vi "Subvi buffer input LUT.vi"(2 "Buffer":refnum<k21>="GALVO1") -> ()   [LabVIEW 2017]
uses:
  GV FIFOIN timeout.vi
  <vilib>/rvi/interface/RandomDataEmulation/niFpgaRandomDataHandleErrors.vi
  <vilib>/rvi/DataTransferAndStorage/Container/Common/niFpgaContainerExecOnDevCompGetState.vi
  <vilib>/rvi/Emulation/niFpgaEmulationIsFPGAContextNoSignature.vi
  <vilib>/rvi/DataTransferAndStorage/Container/Common/niFpgaContainerGetUniqueNameForEmu.vi
  <vilib>/rvi/Emulation/niFpgaProcessEmulError.vi
  <vilib>/rvi/Emulation/niFpgaSctlEmulationGetInTimedLoop.vi
  <vilib>/rvi/errors/nirviReportUnexpectedCaseInternalError (U32).vi
  <vilib>/rvi/Memory/Memory_Emulation/niFpgaMemoryEmulationCacheClearOnFirstRun.vi
  <vilib>/rvi/Memory/Memory_Emulation/nirvimemoryEmulationManagerCache_MakeExclusive.vi
  <vilib>/rvi/Memory/Memory_Emulation/niFpgaMemoryEmulationValidateCache.vi
  <vilib>/rvi/Memory/Memory_Emulation/nirvimemoryEmulationManagerCache_InsertValue.vi
  <vilib>/Utility/error.llb/Clear Errors.vi
  <vilib>/rvi/Memory/Memory_Emulation/nirvimemoryEmulationManagerCache_ReleaseExclusive.vi
  <vilib>/rvi/Memory/Memory_Emulation/nirvimemoryEmulationManagerCache_GetValue.vi
  <vilib>/rvi/Memory/Memory_Emulation/nirvimemoryEmulationManagerCache_SetValue.vi
  <vilib>/rvi/Emulation/niFpgaSctlEmulationResourceMgr.vi
  <vilib>/rvi/DataTransferAndStorage/Container/XNode/niFpgaContainer.xnode
  <vilib>/rvi/interface/RandomDataEmulation/nirviRandomDataFpgaReadWriteTemplate.vi
  <vilib>/rvi/Memory/Memory_Emulation/niFpgaMemoryEmulationRefIn.vi
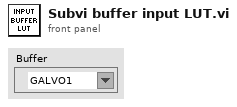
[diagram p1: front panel]
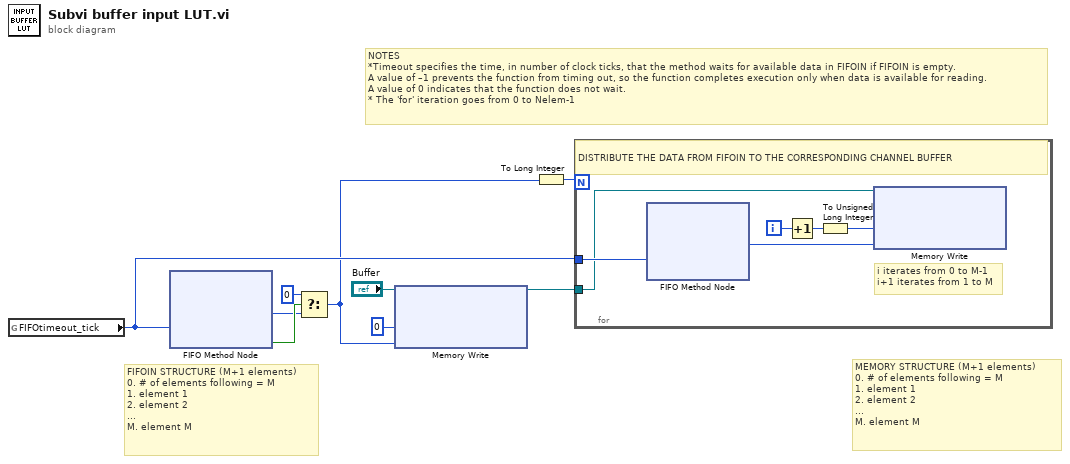
[diagram p0: block diagram]
diagram:
  # "MEMORY STRUCTURE (M+1 elements)\n0. # of elements following = M\n1. element 1\n2. element 2\n...\nM. element M"
  # "FIFOIN STRUCTURE (M+1 elements)\n0. # of elements following = M\n1. element 1\n2. element 2\n...\nM. element M"
  # "NOTES\n*Timeout specifies the time, in number of clock ticks, that the method waits for available data in FIFOIN if FIFOIN is empty.\nA value of –1 prevents the function from timing out, so the function completes execution only when data is available for reading.\nA value of 0 indicates that the function does not wait.\n* The 'for' iteration goes from 0 to Nelem-1"
  n1 = global read "GV FIFOIN timeout.vi" "FIFOtimeout_tick"() -> (w7:i32)
  n2 = xnode ("FIFO Method Node")("Timeout"=w7) -> ("Element"=w5:u32, "Timed Out?"=w6:bool)  [unwired: 1 in, 1 out]
  n3 = Select(t=u32 0, s=w6, f=w5) -> (s? t:f=w3:u32)
  n4 = xnode ("Memory Write")("Address"=u32 0, "Data"=w3, "Memory In"="Buffer") -> ("Memory Out"=w2:refnum<k21>)
  n5 = To Long Integer(number=w3) -> (32bit integer=w8:i32)
  n6 = for {
    N: w8 -> [_]
    tunnel: w7 -> [w15]
    tunnel: w2 -> [w12]
    i -> [w14]
    # "i iterates from 0 to M-1\ni+1 iterates from 1 to M"
    # "DISTRIBUTE THE DATA FROM FIFOIN TO THE CORRESPONDING CHANNEL BUFFER"
    n7 = xnode ("FIFO Method Node")("Timeout"=w15) -> ("Element"=w10:u32)  [unwired: 1 in, 2 out]
    n8 = Increment(x=w14) -> (x+1=w13:i32)
    n9 = To Unsigned Long Integer(number=w13) -> (unsigned 32bit integer=w11:u32)
    n10 = xnode ("Memory Write")("Address"=w11, "Data"=w10, "Memory In"=w12) -> ()  [unwired: 1 out]
  }
